vi "Main.vi"() -> ()   [LabVIEW 2018]
uses:
  <vilib>/Utility/file.llb/Read Delimited Spreadsheet (string).vi
  <vilib>/Utility/file.llb/Write Delimited Spreadsheet (string).vi
panel:
  in  "Done":bool
  in  "configuration file path":path
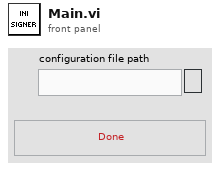
[diagram p1: front panel]
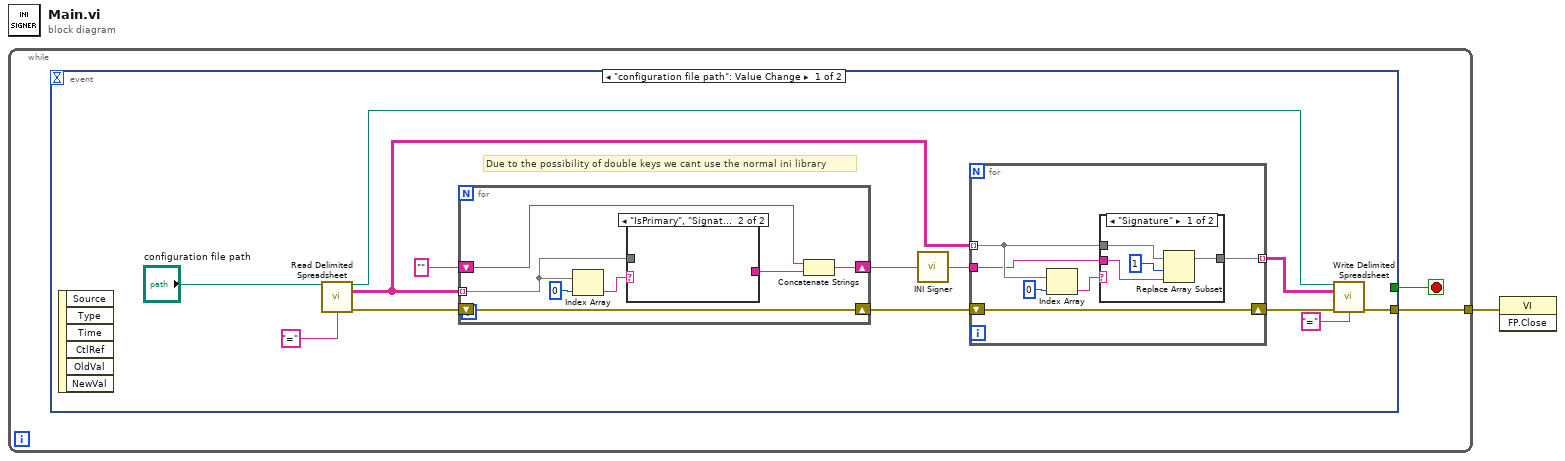
[diagram p0: block diagram]
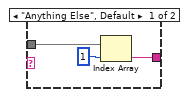
[diagram p3: hidden frame]
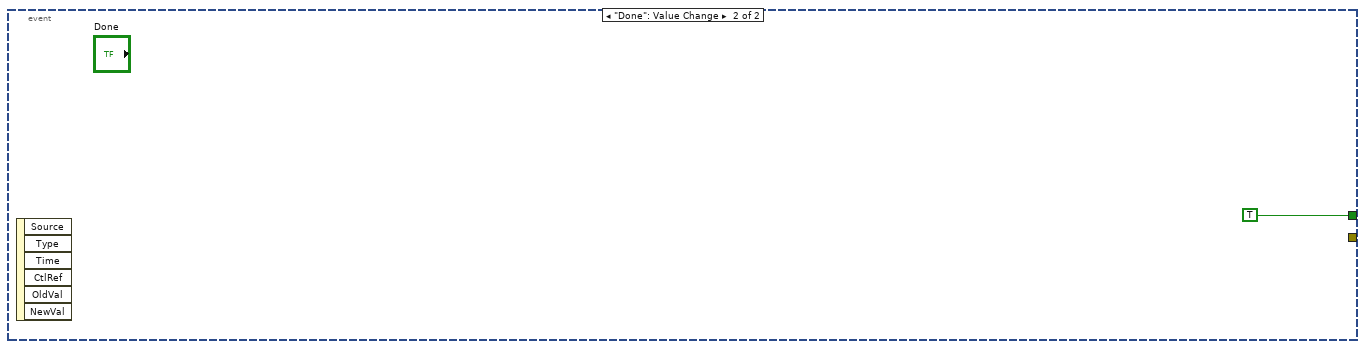
[diagram p4: hidden frame]
diagram:
  n1 = while {
    tunnel: [w2] -> w1
    stop <- w3 stop-if-true
    n2 = event shown="[0] \"configuration file path\": Value Change" {
      selector: _ -> [_ _]
      dyn-events: _ -> [_ _]
      timeout: _ -> [_ _]
      tunnel: [_ TRUE] -> w3
      tunnel: [w4 _] -> w2
      event "configuration file path": Value Change {
        # "Due to the possibility of double keys we cant use the normal ini library"
        n3 = event-data() -> ()  [unwired: 1 in, 6 out]
        n4 = call-poly <vilib>:"Read Delimited Spreadsheet.vi"("file path (dialog if empty)"="configuration file path", "delimiter (\\t)"="=" ("delimiter (\\t)")) -> ("new file path (Not A Path if cancelled)"=w8:path, "all rows"=w11:string[][], "error out"=w14:errorcluster)  [unwired: 8 in, 3 out]
        n5 = for {
          tunnel: w11 -> [w31] mode=indexing
          shift-right: [w29] -> w10
          shift-left: w14 -> [w29]
          shift-right: [w33] -> w12
          shift-left: "" -> [w32]
          n6 = Index Array(array=w31, index=0) -> (element=w28:string)
          n7 = case shown="\"IsPrimary\", \"Signature\"" w28 {
            tunnel: w31 -> [w36 _]
            tunnel: [w35 _] -> w30
            frame "Anything Else", Default {
              n8 = Index Array(array=w36, index=1) -> (element=w35:string)
            }
            frame "IsPrimary", "Signature" {
            }
          }
          n9 = Concatenate Strings(w32, w30) -> (w33:string)
        }
        n10 = call "INI Signer.vi"("String Key Values"=w12) -> ("Signature"=w7:string)
        n11 = for {
          tunnel: w11 -> [w21] mode=indexing
          shift-right: [w20] -> w6
          shift-left: w10 -> [w20]
          tunnel: w7 -> [w18]
          tunnel: [w17] -> w5 mode=indexing
          n12 = Index Array(array=w21, index=0) -> (element=w19:string)
          n13 = case shown="\"Signature\"" w19 {
            tunnel: w21 -> [w26 w27]
            tunnel: w18 -> [w24 _]
            tunnel: [w23 w27] -> w17
            frame "Signature" {
              n14 = Replace Array Subset(array=w26, new element=w24, index=1) -> (w23:string[])
            }
            frame "Anything else", Default {
            }
          }
        }
        n15 = call-poly <vilib>:"Write Delimited Spreadsheet.vi"("file path (dialog if empty)"=w8, "2D data"=w5, "error in (no error)"=w6, "delimiter (\\t)"="=" ("delimiter (\\t)")) -> ("error out"=w4:errorcluster)  [unwired: 10 in, 1 out]
      }
      event "Done": Value Change {
        n16 = event-data() -> ()  [unwired: 1 in, 6 out]
      }
    }
  }
  n17 = invoke class="VI" method="FP.Close"(error in=w1) -> ()  [unwired: 2 in, 3 out]
